vi "unpackReadHighPrec.vi"(4 "长度":i32, 5 "数据":u8[](array[numeric]) format="%.0x") -> (1 "输出参数":T1)   [LabVIEW 2014]
panel:
  out "告警信息":string
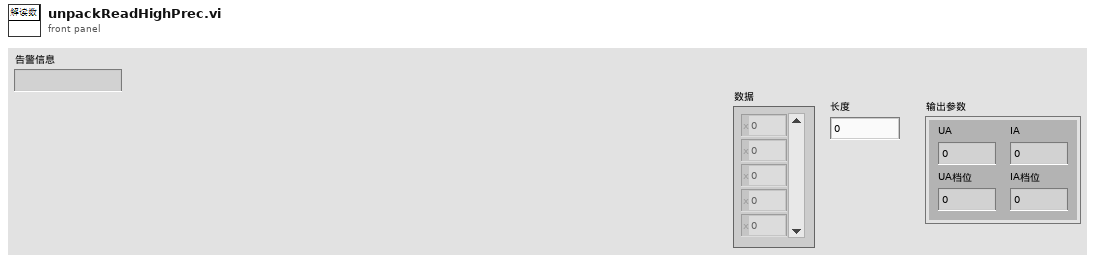
[diagram p1: front panel]
types:
  T1 = cluster{"UA":sgl, "IA":sgl, "UA档位":sgl, "IA档位":sgl}
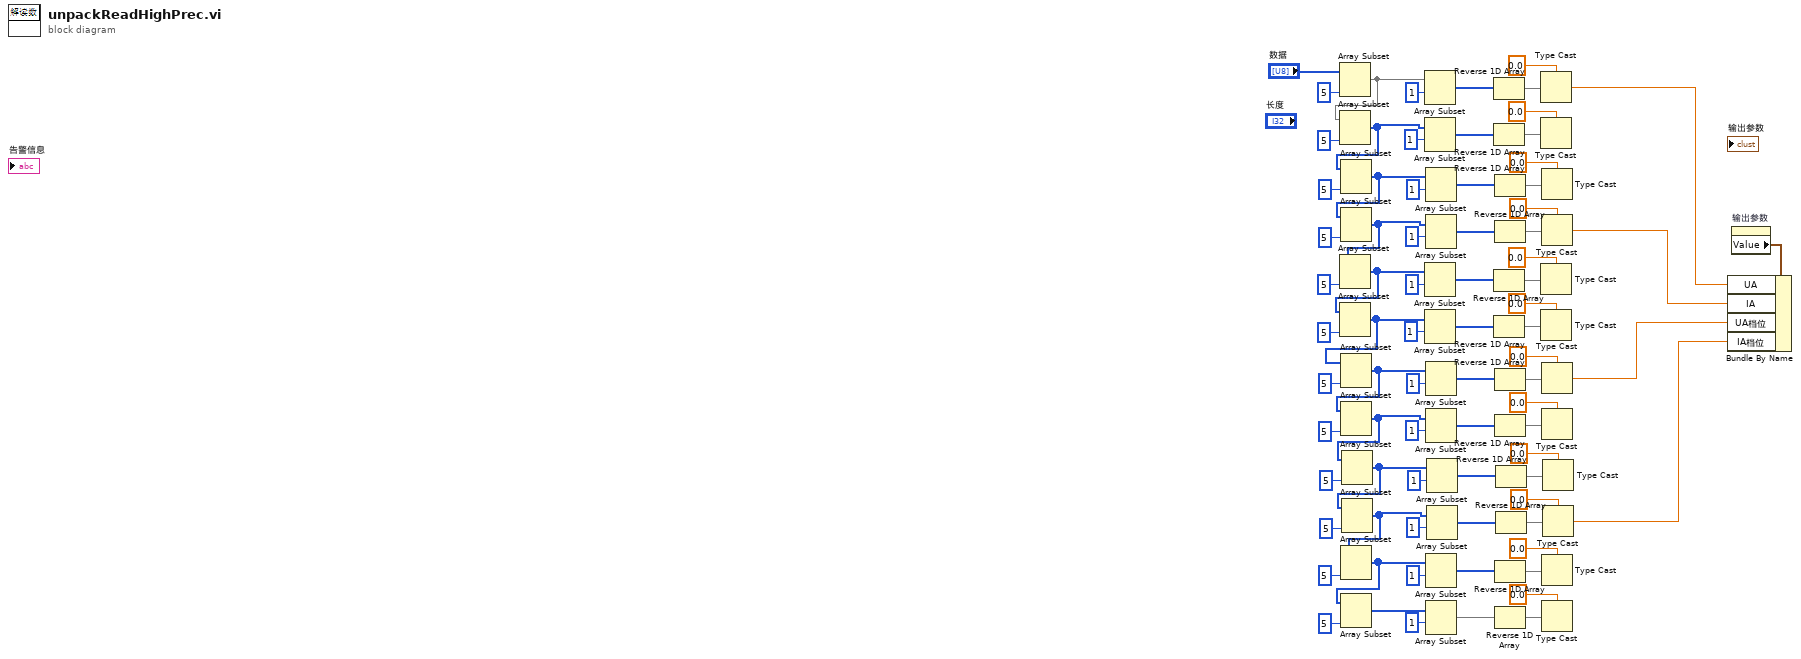
[diagram p0: block diagram]
diagram:
  n1 = Array Subset(array="数据", length=5 ("长度")) -> (w78:u8[])  [unwired: 1 in]
  n2 = Array Subset(array=w78, length=5 ("长度")) -> (w43:u8[])  [unwired: 1 in]
  n3 = Array Subset(array=w43, length=5 ("长度")) -> (w55:u8[])  [unwired: 1 in]
  n4 = Array Subset(array=w55, length=5 ("长度")) -> (w42:u8[])  [unwired: 1 in]
  n5 = Array Subset(array=w42, length=5 ("长度")) -> (w54:u8[])  [unwired: 1 in]
  n6 = Array Subset(array=w54, length=5 ("长度")) -> (w7:u8[])  [unwired: 1 in]
  n7 = Array Subset(array=w7, length=5 ("长度")) -> (w8:u8[])  [unwired: 1 in]
  n8 = Array Subset(array=w8, length=5 ("长度")) -> (w6:u8[])  [unwired: 1 in]
  n9 = Array Subset(array=w6, length=5 ("长度")) -> (w29:u8[])  [unwired: 1 in]
  n10 = Array Subset(array=w29, length=5 ("长度")) -> (w5:u8[])  [unwired: 1 in]
  n11 = Array Subset(array=w5, length=5 ("长度")) -> (w30:u8[])  [unwired: 1 in]
  n12 = Array Subset(array=w30, length=5 ("长度")) -> (w31:u8[])  [unwired: 1 in]
  n13 = Array Subset(array=w78, index=1 ("索引")) -> (w75:u8[])  [unwired: 1 in]
  n14 = Array Subset(array=w43, index=1 ("长度")) -> (w72:u8[])  [unwired: 1 in]
  n15 = Array Subset(array=w54, index=1 ("索引")) -> (w51:u8[])  [unwired: 1 in]
  n16 = Array Subset(array=w7, index=1 ("长度")) -> (w48:u8[])  [unwired: 1 in]
  n17 = Array Subset(array=w55, index=1 ("索引")) -> (w58:u8[])  [unwired: 1 in]
  n18 = Array Subset(array=w42, index=1 ("长度")) -> (w61:u8[])  [unwired: 1 in]
  n19 = Array Subset(array=w8, index=1 ("索引")) -> (w11:u8[])  [unwired: 1 in]
  n20 = Array Subset(array=w6, index=1 ("长度")) -> (w14:u8[])  [unwired: 1 in]
  n21 = Array Subset(array=w30, index=1 ("索引")) -> (w34:u8[])  [unwired: 1 in]
  n22 = Array Subset(array=w31, index=1 ("长度")) -> (w37:u8[])  [unwired: 1 in]
  n23 = Array Subset(array=w29, index=1 ("索引")) -> (w26:u8[])  [unwired: 1 in]
  n24 = Array Subset(array=w5, index=1 ("长度")) -> (w23:u8[])  [unwired: 1 in]
  n25 = Reverse 1D Array(array=w75) -> (reversed array=w76:u8[])
  n26 = Reverse 1D Array(array=w72) -> (reversed array=w74:u8[])
  n27 = Reverse 1D Array(array=w51) -> (reversed array=w52:u8[])
  n28 = Reverse 1D Array(array=w48) -> (reversed array=w50:u8[])
  n29 = Reverse 1D Array(array=w58) -> (reversed array=w57:u8[])
  n30 = Reverse 1D Array(array=w61) -> (reversed array=w59:u8[])
  n31 = Reverse 1D Array(array=w11) -> (reversed array=w10:u8[])
  n32 = Reverse 1D Array(array=w14) -> (reversed array=w12:u8[])
  n33 = Reverse 1D Array(array=w34) -> (reversed array=w33:u8[])
  n34 = Reverse 1D Array(array=w37) -> (reversed array=w35:u8[])
  n35 = Reverse 1D Array(array=w26) -> (reversed array=w27:u8[])
  n36 = Reverse 1D Array(array=w23) -> (reversed array=w25:u8[])
  n37 = Type Cast(type=sgl 0.0, x=w76) -> (*(type *) &x=w4:sgl)
  n38 = Type Cast(type=sgl 0.0, x=w74) -> ()  [unwired: 1 out]
  n39 = Type Cast(type=sgl 0.0, x=w52) -> ()  [unwired: 1 out]
  n40 = Type Cast(type=sgl 0.0, x=w50) -> ()  [unwired: 1 out]
  n41 = Type Cast(type=sgl 0.0, x=w57) -> ()  [unwired: 1 out]
  n42 = Type Cast(type=sgl 0.0, x=w59) -> (*(type *) &x=w3:sgl)
  n43 = Type Cast(type=sgl 0.0, x=w10) -> (*(type *) &x=w2:sgl)
  n44 = Type Cast(type=sgl 0.0, x=w12) -> ()  [unwired: 1 out]
  n45 = Type Cast(type=sgl 0.0, x=w33) -> ()  [unwired: 1 out]
  n46 = Type Cast(type=sgl 0.0, x=w35) -> ()  [unwired: 1 out]
  n47 = Type Cast(type=sgl 0.0, x=w27) -> ()  [unwired: 1 out]
  n48 = Type Cast(type=sgl 0.0, x=w25) -> (*(type *) &x=w1:sgl)
  n49 = property on="输出参数" class="Clust (严格)"() -> ("Value"=w70:T1)  [unwired: 2 in, 2 out]
  n50 = Bundle By Name(cluster=w70, "UA"=w4, "IA"=w3, "UA档位"=w2, "IA档位"=w1) -> ()  [unwired: 1 out]
